vi "programa 4 segund parcial array.vi"() -> ()   [LabVIEW 2011]
panel:
  out "Array":dbl[](array[numeric])
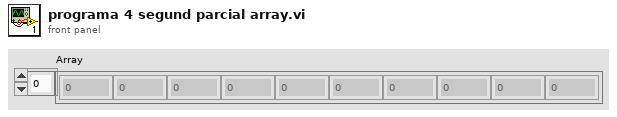
[diagram p1: front panel]
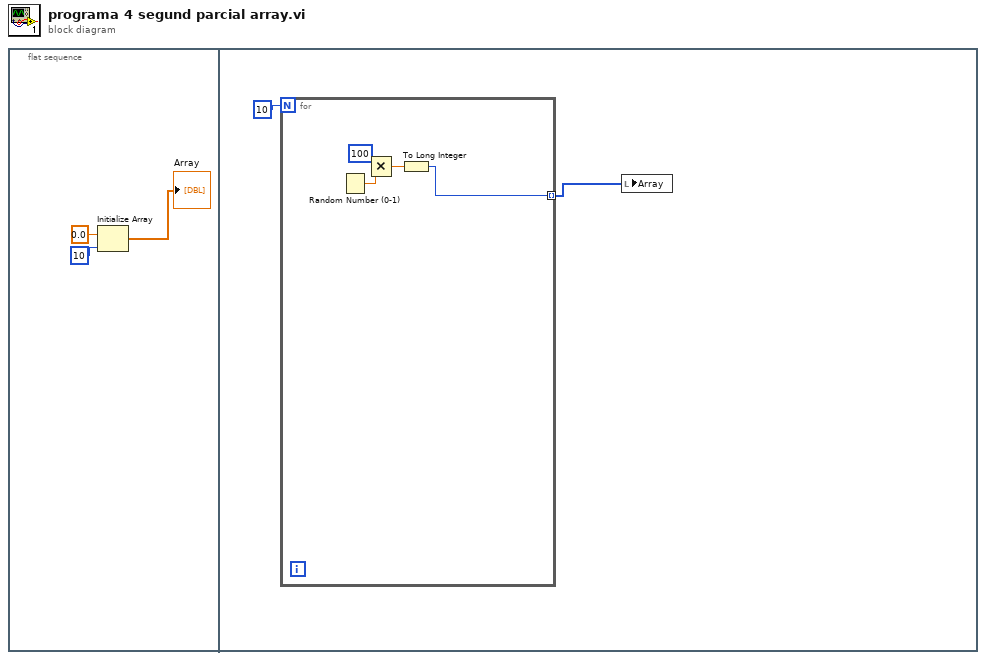
[diagram p0: block diagram]
diagram:
  n1 = flat-sequence {
    frame #0 {
      n2 = Initialize Array(0.0 ("element"), 10) -> (→"Array":dbl[])
    }
    frame #1 {
      n3 = for {
        N: 10 -> [_]
        tunnel: [w6] -> w4 mode=indexing
        n4 = Random Number (0-1)() -> (number: 0 to 1=w9:dbl)
        n5 = Multiply(x=100, y=w9) -> (x*y=w7:dbl)
        n6 = To Long Integer(number=w7) -> (32bit integer=w6:i32)
      }
      n7 = local write "Array"(w4) -> ()
    }
  }
